vi "VisionExecute.v.vi"   [LabVIEW 2023]
uses:
  <vilib>/Rock Robotics/WPI/ThirdParty/JAS_Junk/TrajLib/Trajectory_Library.lvlib
  <vilib>/Rock Robotics/WPI/ThirdParty/PhotonVisionLib/PhotonVisionLib.lvlib
  <vilib>/Rock Robotics/WPI/ThirdParty/PhotonVisionLib/Enum/PhotonPoseStrategy_ENUM.ctl
  VisionGlobal.vi
  <vilib>/Rock Robotics/WPI/ThirdParty/JAS_Junk/TrajLib/TypeDef/TRANSLATION2D.ctl
  <vilib>/Rock Robotics/WPI/ThirdParty/JAS_Junk/TrajLib/TypeDef/ROTATION2D.ctl
  <vilib>/Rock Robotics/WPI/ThirdParty/JAS_Junk/TrajLib/TypeDef/POSE2D.ctl
  VisionNetworkingGlobal.vi
  <vilib>/Rock Robotics/Network Tables/NT Write Number.vi
  <vilib>/Rock Robotics/WPI/ThirdParty/JAS_Junk/TrajLib/VI/AprilTagFieldLayout_New2024.vi
types:
  T1 = typedef "PhotonVisionLib.lvlib/PhotonPoseStrategy_ENUM.ctl" = enum16{"LOWEST_AMBIGUITY", "CLOSEST_TO_CAMERA_HEIGHT", "CLOSEST_TO_REFERENCE_POSE", "CLOSEST_TO_LAST_POSE", "AVERAGE_BEST_TARGETS", "MULTI_TAG_PNP_ON_COPROCESSOR", "MULTI_TAG_PNP_ON_RIO"}
  T2 = typedef "Trajectory_Library.lvlib/TRANSLATION3D.ctl" = cluster{"X":dbl, "Y":dbl, "Z":dbl}
  T3 = typedef "Trajectory_Library.lvlib/ROTATION3D.ctl" = cluster{"Q_quaternion":T4}
  T4 = typedef "Trajectory_Library.lvlib/QUATERNION.ctl" = cluster{"R":dbl, "V":dbl[]}
  T5 = typedef "Trajectory_Library.lvlib/TRANSFORM3D.ctl" = cluster{"TRANSLATION3D":T2, "ROTATION3D":T3, "XF":bool}
  T6 = typedef "PhotonVisionLib.lvlib/PhotonPipelineResultType.ctl" = cluster{"Targets":T7[], "PhotonMultiTargetPNPResult":T9, "PhotonPipelineMetadata":T11}
  T7 = typedef "PhotonVisionLib.lvlib/PhotonTrackedTargetType.ctl" = cluster{"Yaw":dbl, "Pitch":dbl, "Area":dbl, "Skew":dbl, "MinAreaRectCorners":T8[], "BestCameraToTarget":T5, "FiducialId":i32, "AltCameraToTarget":T5, "PoseAmbiguity":dbl, "DetectedCorners":T8[], "ObjDetectId":i32, "ObjDetectConf":sgl}
  T8 = typedef "PhotonVisionLib.lvlib/TargetCornerType.ctl" = cluster{"X":dbl, "Y":dbl}
  T9 = typedef "PhotonVisionLib.lvlib/PhotonMultiTargetPNPResultType.ctl" = cluster{"PhotonPNPResult":T10, "FiducialIDsUsed":i16[]}
  T10 = typedef "PhotonVisionLib.lvlib/PhotonPNPResultType.ctl" = cluster{"IsPresent":bool, "bestReprojErr":dbl, "altReprojErr":dbl, "ambiguity":dbl, "Best":T5, "Alt":T5}
  T11 = typedef "PhotonVisionLib.lvlib/PhotonPipelineMetadataType.ctl" = cluster{"CaptureTimestampMicros":i64, "PublishTimestampMicros":i64, "SequenceID":i64, "TimeSinceLastPong":i64}
  T12 = typedef "Trajectory_Library.lvlib/AprilTagFieldLayout.ctl" = cluster{"AprilTagMap":map{i32, T13}, "FieldLength":dbl, "FieldWidth":dbl, "OriginPosition ":T15, "OriginPose3d":T14}
  T13 = typedef "Trajectory_Library.lvlib/AprilTag.ctl" = cluster{"ID":i32, "POSE3D":T14}
  T14 = typedef "Trajectory_Library.lvlib/POSE3D.ctl" = cluster{"Translation3d":T2, "Rotation3d":T3}
  T15 = typedef "Trajectory_Library.lvlib/AprilTagFieldLayoutOrignPosition_ENUM.ctl" = enum16{"kBlueAllianceWallRightSide,", "kRedAllianceWallRightSide,"}
  T16 = typedef "Trajectory_Library.lvlib/POSE2D.ctl" = cluster{"TRANSLATION":T17, "ROTATION":T18}
  T17 = typedef "Trajectory_Library.lvlib/TRANSLATION2D.ctl" = cluster{"X":dbl, "Y":dbl}
  T18 = typedef "Trajectory_Library.lvlib/ROTATION2D.ctl" = cluster{"VALUE":dbl, "COS":dbl, "SIN":dbl}
  T19 = typedef "PhotonVisionLib.lvlib/PhotonPoseEstimator_Configuration.ctl" = cluster{"Primary Strategy":T1, "Camera":string, "Initial Pose":T14, "HighestAmbiguity":dbl, "RobotToCamera":T5, "FallBack Strategy":T1, "BaseNTName":string}
  T20 = typedef "Trajectory_Library.lvlib/SWERVE_DRIVE_KINEMATICS.ctl" = cluster{"NumModules":i32, "InverseKinematics":T21, "ForwardKinematics":T21, "Modules":T17[], "PrevCoR":T17, "SavedModuleStates":T22[]}
  T21 = typedef "NI_Matrix.lvlib/RealMatrix.ctl" = dbl[][]
  T22 = typedef "Trajectory_Library.lvlib/SWERVE_DRIVE_MODULE_STATE.ctl" = cluster{"Speed":dbl, "Angle":T18}
  T23 = typedef "Trajectory_Library.lvlib/SWERVE_DRIVE_MODULE_POSITION.ctl" = cluster{"Distance":dbl, "Angle":T18, "P":bool}
  T24 = typedef "Trajectory_Library.lvlib/SWERVE_DRIVE_POSE_EST2_CONFIG.ctl" = cluster{"Wheel_Locations M":T17[], "Odom X std dev M":dbl, "Odom Y std dev M":dbl, "Odom Heading std dev Rad":dbl, "Vision X std dev M":dbl, "Vision Y std dev M":dbl, "Vision Heading std dev Rad":dbl}
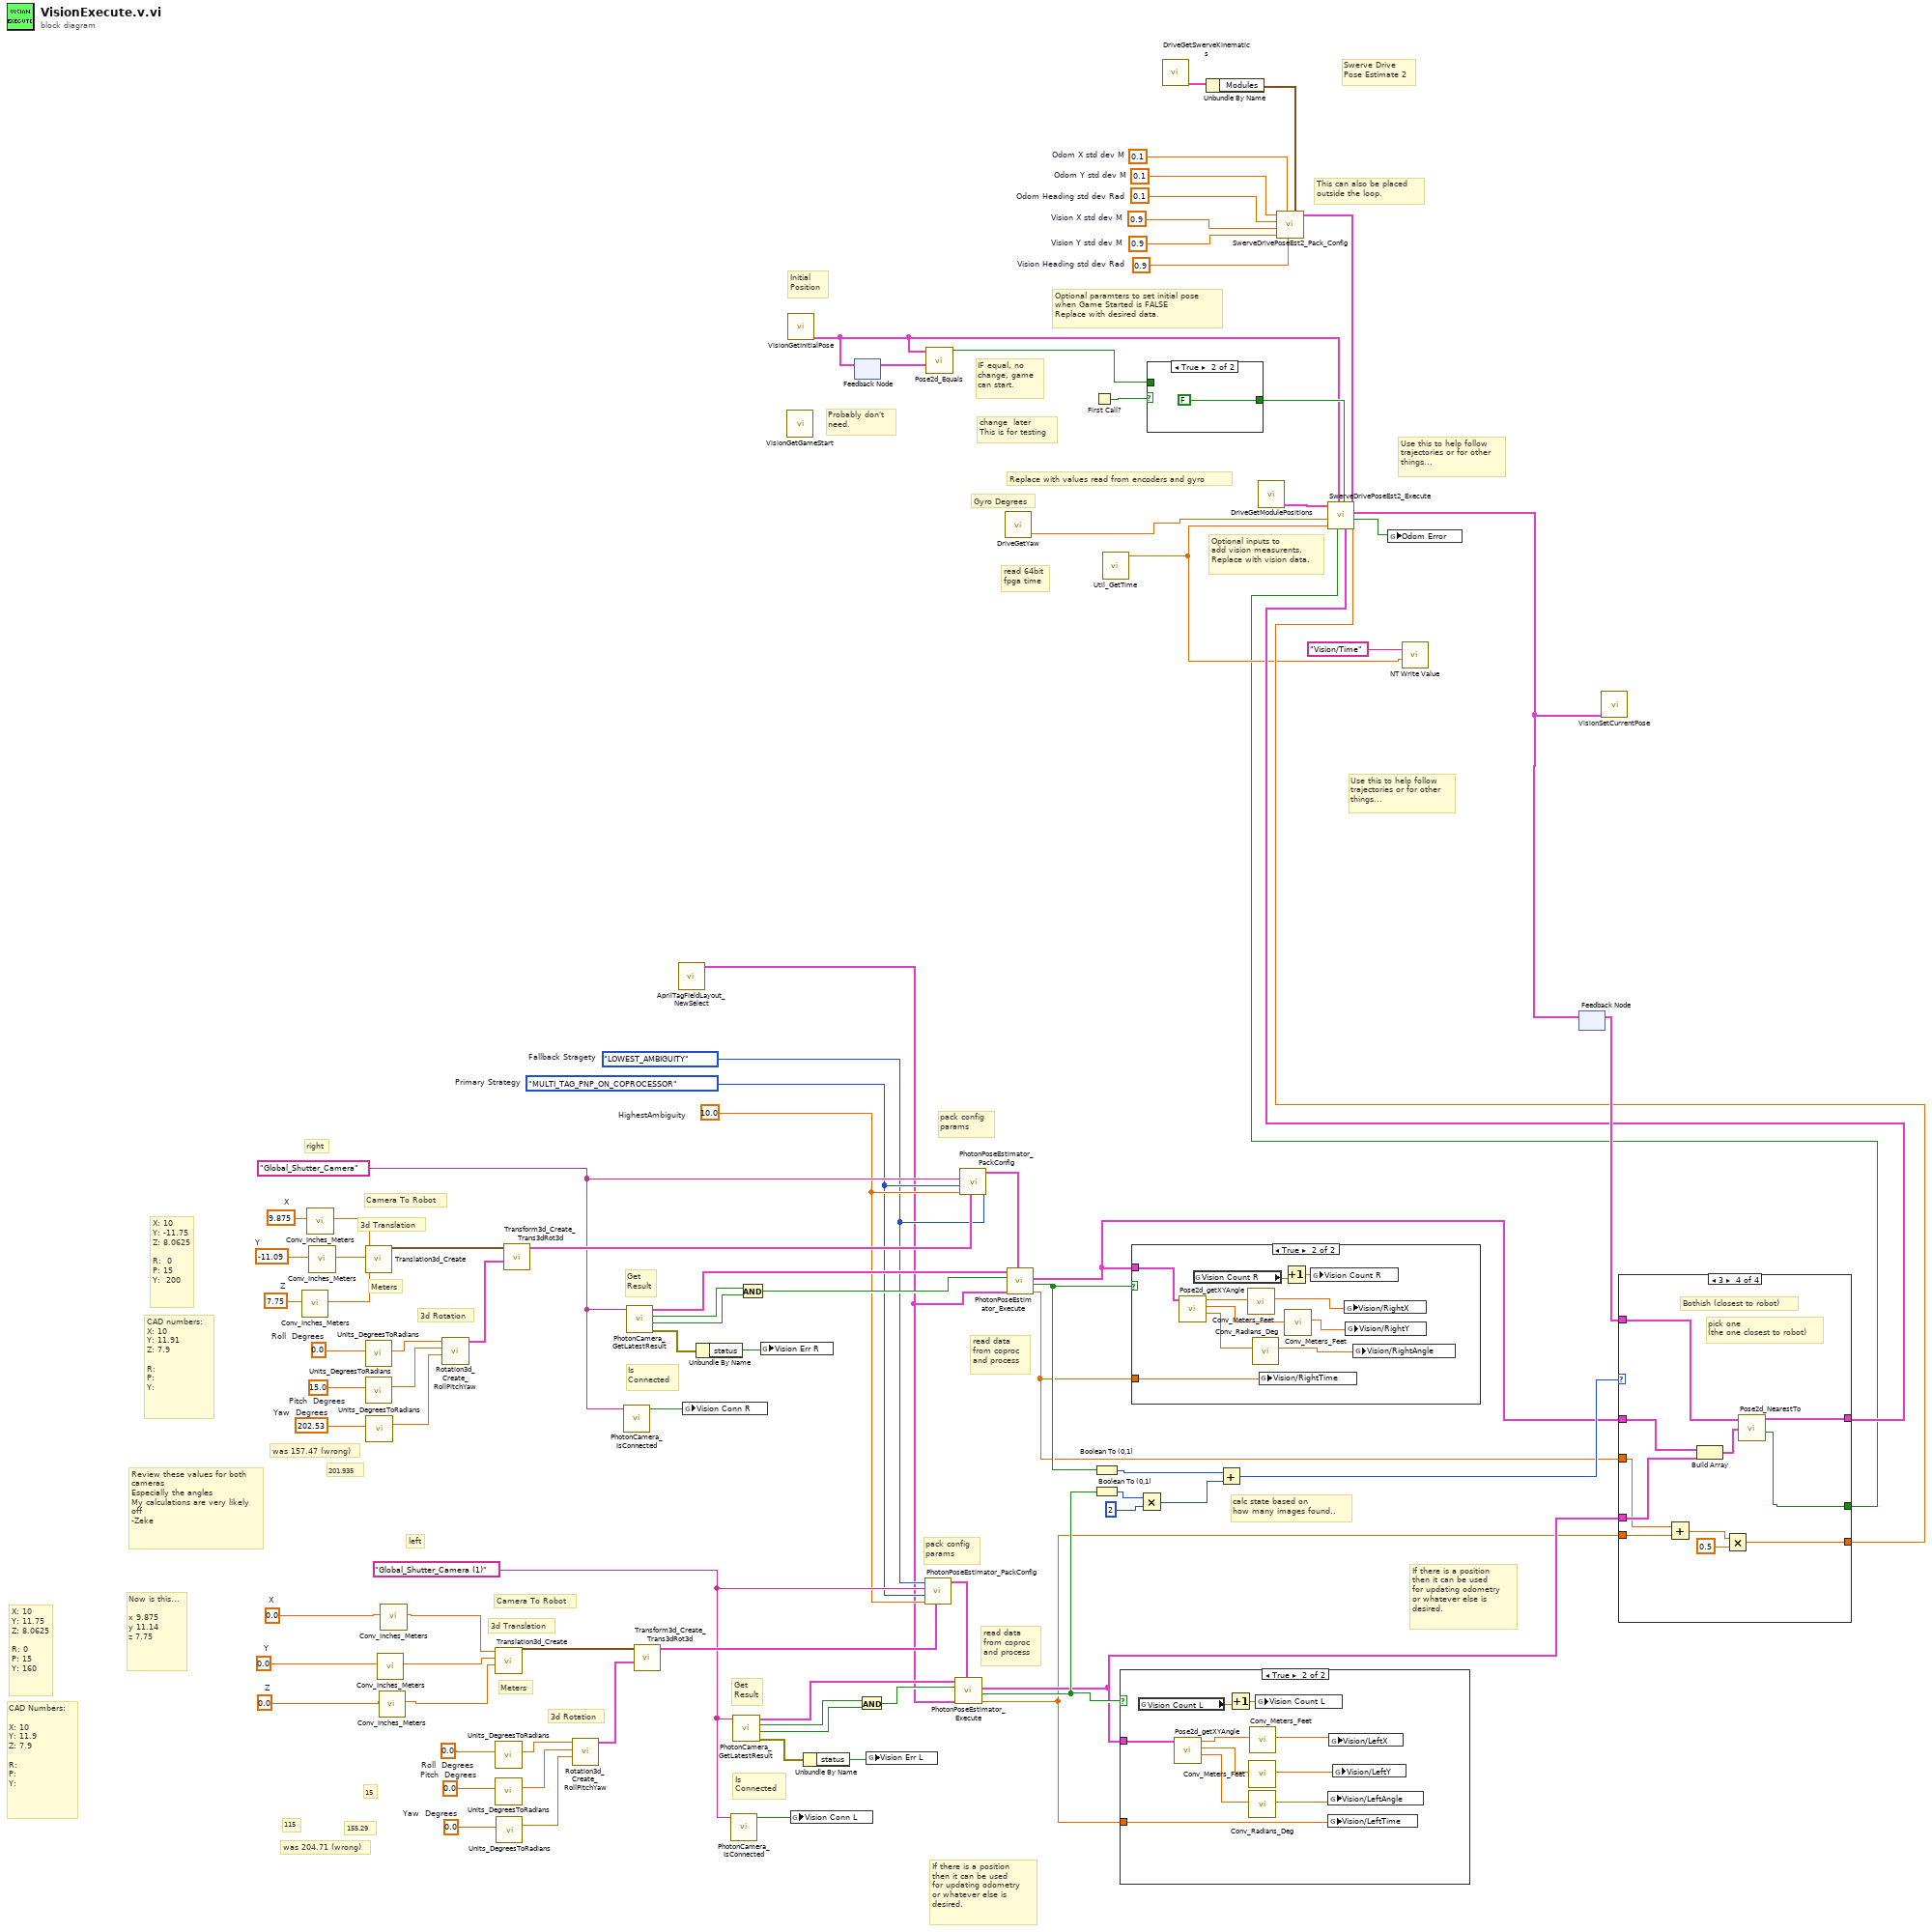
[diagram p0: block diagram]
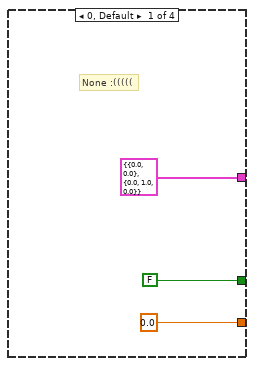
[diagram p3: hidden frame]
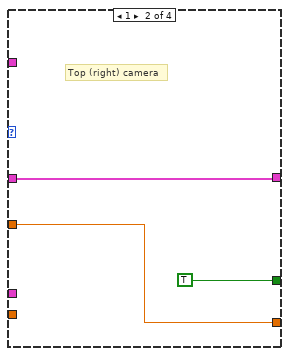
[diagram p4: hidden frame]
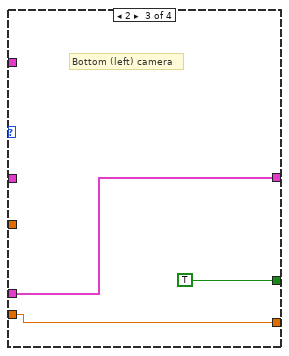
[diagram p5: hidden frame]
diagram:
  w14 = PhotonPoseStrategy_ENUM."LOWEST_AMBIGUITY"  # Fallback Stragety
  w24 = 0.1  # Odom Y std dev M
  w25 = 0.1  # Odom Heading std dev Rad
  w26 = 0.9  # Vision X std dev M
  w27 = 0.9  # Vision Y std dev M
  w28 = 0.1  # Odom X std dev M
  w29 = 0.9  # Vision Heading std dev Rad
  w62 = 0.0  # Roll  Degrees
  w61 = 0.0  # Pitch  Degrees
  w60 = 0.0  # Yaw  Degrees
  w47 = 0.0  # Z
  w51 = 0.0  # X
  w49 = 0.0  # Y
  w56 = "Global_Shutter_Camera (1)" ("CameraName")
  w80 = 0.0  # Roll  Degrees
  w79 = 15.0  # Pitch  Degrees
  w78 = 202.53  # Yaw  Degrees
  w41 = 7.75  # Z
  w45 = 9.875  # X
  w43 = -11.09  # Y
  w39 = 10.0  # HighestAmbiguity
  w38 = PhotonPoseStrategy_ENUM."MULTI_TAG_PNP_ON_COPROCESSOR"  # Primary Strategy
  w74 = "Global_Shutter_Camera" ("CameraName")
  # "calc state based on\nhow many images found.."
  # "read data\nfrom coproc\nand process"
  # "read data\nfrom coproc\nand process"
  # "pack config\nparams"
  # "pack config\nparams"
  # "15"
  # "155.29"
  # "Now is this...\n\nx 9.875\ny 11.14\nz 7.75"
  # "115"
  # "was 157.47 (wrong)"
  # "was 204.71 (wrong)"
  # "CAD Numbers:\n\nX: 10 \nY: 11.9\nZ: 7.9\n\nR:\nP:\nY:"
  # "CAD numbers:\nX: 10\nY: 11.91\nZ: 7.9\n\nR:\nP:\nY:"
  # "X: 10\nY: 11.75\nZ: 8.0625\n\nR: 0\nP: 15\nY: 160"
  # "X: 10 \nY: -11.75\nZ: 8.0625\n\nR:  0\nP: 15\nY:  200"
  # "Probably don't\nneed."
  # "IF equal, no \nchange, game\ncan start."
  # "Initial\nPosition"
  # "201.935"
  # "change  later\nThis is for testing"
  # "Review these values for both cameras\nEspecially the angles\nMy calculations are very likely off\n-Zeke"
  # "Optional inputs to\nadd vision measurents.\nReplace with vision data."
  # "Replace with values read from encoders and gyro"
  # "Optional paramters to set initial pose\nwhen Game Started is FALSE\nReplace with desired data."
  # "read 64bit\nfpga time"
  # "This can also be placed \noutside the loop."
  # "Use this to help follow\ntrajectories or for other\nthings..."
  # "Swerve Drive \nPose Estimate 2"
  # "Use this to help follow\ntrajectories or for other\nthings..."
  # "right"
  # "left"
  # "If there is a position\nthen it can be used\nfor updating odometry\nor whatever else is \ndesired."
  # "Meters"
  # "Camera To Robot"
  # "3d Rotation"
  # "3d Translation"
  # "Is\nConnected"
  # "Get\nResult"
  # "If there is a position\nthen it can be used\nfor updating odometry\nor whatever else is \ndesired."
  # "Meters"
  # "Camera To Robot"
  # "3d Rotation"
  # "3d Translation"
  # "Is\nConnected"
  # "Get\nResult"
  # "Gyro Degrees"
  n1 = call <vilib>:"Conv_Inches_Meters.vi"("INCH"=w41) -> ("Meters"=w40:dbl)  [unwired: 10 in]
  n2 = call <vilib>:"Conv_Inches_Meters.vi"("INCH"=w45) -> ("Meters"=w44:dbl)  [unwired: 10 in]
  n3 = call <vilib>:"Conv_Inches_Meters.vi"("INCH"=w43) -> ("Meters"=w42:dbl)  [unwired: 10 in]
  n4 = call <vilib>:"Translation3d_Create.vi"("Z"=w40, "Y"=w42, "X"=w44) -> ("TRANSLATION3D"=w81:T2)  [unwired: 8 in]
  n5 = call <vilib>:"Units_DegreesToRadians.vi"("Degrees"=w80) -> ("Radians"=w77:dbl)  [unwired: 10 in]
  n6 = call <vilib>:"Units_DegreesToRadians.vi"("Degrees"=w79) -> ("Radians"=w76:dbl)  [unwired: 10 in]
  n7 = call <vilib>:"Units_DegreesToRadians.vi"("Degrees"=w78) -> ("Radians"=w75:dbl)  [unwired: 10 in]
  n8 = call <vilib>:"Conv_Inches_Meters.vi"("INCH"=w49) -> ("Meters"=w48:dbl)  [unwired: 10 in]
  n9 = call <vilib>:"Conv_Inches_Meters.vi"("INCH"=w47) -> ("Meters"=w46:dbl)  [unwired: 10 in]
  n10 = call <vilib>:"Conv_Inches_Meters.vi"("INCH"=w51) -> ("Meters"=w50:dbl)  [unwired: 10 in]
  n11 = call <vilib>:"Rotation3d_Create_RollPitchYaw.vi"("Yaw"=w75, "Pitch"=w76, "Roll"=w77) -> ("Rotation3d"=w82:T3)  [unwired: 8 in]
  n12 = call <vilib>:"Translation3d_Create.vi"("Z"=w46, "Y"=w48, "X"=w50) -> ("TRANSLATION3D"=w63:T2)  [unwired: 8 in]
  n13 = call <vilib>:"Units_DegreesToRadians.vi"("Degrees"=w62) -> ("Radians"=w59:dbl)  [unwired: 10 in]
  n14 = call <vilib>:"Units_DegreesToRadians.vi"("Degrees"=w61) -> ("Radians"=w58:dbl)  [unwired: 10 in]
  n15 = call <vilib>:"Units_DegreesToRadians.vi"("Degrees"=w60) -> ("Radians"=w57:dbl)  [unwired: 10 in]
  n16 = call <vilib>:"Transform3d_Create_Trans3dRot3d.vi"("Rotation3d"=w82, "Translation3d"=w81) -> ("Transform3d"=w83:T5)  [unwired: 9 in]
  n17 = call <vilib>:"Rotation3d_Create_RollPitchYaw.vi"("Yaw"=w57, "Pitch"=w58, "Roll"=w59) -> ("Rotation3d"=w64:T3)  [unwired: 8 in]
  n18 = call <vilib>:"PhotonCamera_IsConnected.vi"("CameraName"=w74) -> ("IsConnected"=w72:bool)  [unwired: 9 in, 1 out]
  n19 = call <vilib>:"PhotonCamera_GetLatestResult.vi"("CameraName"=w74) -> ("error out"=w71:errorcluster, "New Data"=w87:bool, "HasTargets"=w86:bool, "PipelineResult"=w84:T6)  [unwired: 6 in, 1 out]
  n20 = call <vilib>:"Transform3d_Create_Trans3dRot3d.vi"("Rotation3d"=w64, "Translation3d"=w63) -> ("Transform3d"=w65:T5)  [unwired: 9 in]
  n21 = call-poly <vilib>:"AprilTagFieldLayout_NewSelect.vi"() -> ("AprilTagFieldLayout"=w1:T12)  [unwired: 11 in]
  n22 = global write "VisionGlobal.vi" "Vision Conn R"(w72) -> ()
  n23 = Unbundle By Name(w71) -> ("status"=w70:bool)
  n24 = call <vilib>:"PhotonCamera_IsConnected.vi"("CameraName"=w56) -> ("IsConnected"=w54:bool)  [unwired: 9 in, 1 out]
  n25 = call <vilib>:"PhotonCamera_GetLatestResult.vi"("CameraName"=w56) -> ("error out"=w53:errorcluster, "New Data"=w69:bool, "HasTargets"=w68:bool, "PipelineResult"=w66:T6)  [unwired: 6 in, 1 out]
  n26 = And(x=w86, y=w87) -> (x .and. y?=w85:bool)
  n27 = global write "VisionGlobal.vi" "Vision Err R"(w70) -> ()
  n28 = call "VisionGetGameStart.vi"() -> ()  [unwired: 11 in, 1 out]
  n29 = call "VisionGetInitialPose.vi"() -> ("InitialPose"=w4:T16)  [unwired: 10 in]
  n30 = global write "VisionGlobal.vi" "Vision Conn L"(w54) -> ()
  n31 = Unbundle By Name(w53) -> ("status"=w52:bool)
  n32 = feedback-in #1(w4) -> ()
  n33 = feedback #1() -> (w3:T16)  [unwired: 1 in]
  n34 = And(x=w68, y=w69) -> (x .and. y?=w67:bool)
  n35 = global write "VisionGlobal.vi" "Vision Err L"(w52) -> ()
  n36 = call <vilib>:"PhotonPoseEstimator_PackConfig.vi"("FallBack Strategy"=w14, "RobotToCamera"=w65, "HighestAmbiguity"=w39, "PirmaryStrategy"=w38, "Camera"=w56) -> ("PoseEstimator_Configuration"=w55:T19)  [unwired: 6 in]
  n37 = call <vilib>:"Pose2d_Equals.vi"("other POSE"=w3, "in POSE"=w4) -> ("Equals"=w2:bool)  [unwired: 9 in]
  n38 = call <vilib>:"PhotonPoseEstimator_Execute.vi"("Configuration"=w55, "AprilTagFieldLayout"=w1, "PIpeline Has \nNew Results"=w67, "PipelineResult"=w66) -> ("TimeStamp_Seconds"=w9:dbl, "New Pose Found"=w36:bool, "EstimatedPose2d"=w11:T16)  [unwired: 1 in, 4 out]
  n39 = call <vilib>:"PhotonPoseEstimator_PackConfig.vi"("FallBack Strategy"=w14, "RobotToCamera"=w83, "HighestAmbiguity"=w39, "PirmaryStrategy"=w38, "Camera"=w74) -> ("PoseEstimator_Configuration"=w73:T19)  [unwired: 6 in]
  n40 = call "DriveGetYaw.vi"() -> ("Yaw"=w19:dbl)  [unwired: 11 in]
  n41 = call <vilib>:"PhotonPoseEstimator_Execute.vi"("Configuration"=w73, "AprilTagFieldLayout"=w1, "PIpeline Has \nNew Results"=w85, "PipelineResult"=w84) -> ("TimeStamp_Seconds"=w8:dbl, "New Pose Found"=w37:bool, "EstimatedPose2d"=w10:T16)  [unwired: 1 in, 4 out]
  n42 = First Call?() -> (First Call?: T/F=w12:bool)
  n43 = Boolean To (0,1)(Boolean=w37) -> (0, 1=w32:i16)
  n44 = Boolean To (0,1)(Boolean=w36) -> (0, 1=w35:i16)
  n45 = call <vilib>:"Util_GetTime.vi"() -> ("FPGA_Time_Seconds"=w6:dbl)  [unwired: 9 in, 2 out]
  n46 = case shown="True" w36 {
    tunnel: w11 -> [_ w95]
    tunnel: w9 -> [_ w94]
    frame False {
    }
    frame True {
      n47 = global read "VisionGlobal.vi" "Vision Count L"() -> (w96:dbl)
      n48 = call <vilib>:"Pose2d_getXYAngle.vi"("in POSE"=w95) -> ("Angle"=w89:dbl, "Y"=w91:dbl, "X"=w93:dbl)  [unwired: 8 in]
      n49 = Increment(x=w96) -> (x+1=w97:dbl)
      n50 = call <vilib>:"Conv_Meters_Feet.vi"("Meters"=w91) -> ("Feet"=w90:dbl)  [unwired: 10 in]
      n51 = call <vilib>:"Conv_Radians_Deg.vi"("Radians"=w89) -> ("Degrees"=w88:dbl)  [unwired: 10 in]
      n52 = call <vilib>:"Conv_Meters_Feet.vi"("Meters"=w93) -> ("Feet"=w92:dbl)  [unwired: 10 in]
      n53 = global write "VisionGlobal.vi" "Vision Count L"(w97) -> ()
      n54 = global write "VisionNetworkingGlobal.vi" "Vision/LeftAngle"(w88) -> ()
      n55 = global write "VisionNetworkingGlobal.vi" "Vision/LeftTime"(w94) -> ()
      n56 = global write "VisionNetworkingGlobal.vi" "Vision/LeftX"(w92) -> ()
      n57 = global write "VisionNetworkingGlobal.vi" "Vision/LeftY"(w90) -> ()
    }
  }
  n58 = case shown="True" w37 {
    tunnel: w10 -> [_ w105]
    tunnel: w8 -> [_ w104]
    frame False {
    }
    frame True {
      n59 = call <vilib>:"Pose2d_getXYAngle.vi"("in POSE"=w105) -> ("Angle"=w99:dbl, "Y"=w101:dbl, "X"=w103:dbl)  [unwired: 8 in]
      n60 = global read "VisionGlobal.vi" "Vision Count R"() -> (w106:dbl)
      n61 = call <vilib>:"Conv_Meters_Feet.vi"("Meters"=w103) -> ("Feet"=w102:dbl)  [unwired: 10 in]
      n62 = call <vilib>:"Conv_Radians_Deg.vi"("Radians"=w99) -> ("Degrees"=w98:dbl)  [unwired: 10 in]
      n63 = global write "VisionNetworkingGlobal.vi" "Vision/RightTime"(w104) -> ()
      n64 = Increment(x=w106) -> (x+1=w107:dbl)
      n65 = call <vilib>:"Conv_Meters_Feet.vi"("Meters"=w101) -> ("Feet"=w100:dbl)  [unwired: 10 in]
      n66 = global write "VisionGlobal.vi" "Vision Count R"(w107) -> ()
      n67 = global write "VisionNetworkingGlobal.vi" "Vision/RightX"(w102) -> ()
      n68 = global write "VisionNetworkingGlobal.vi" "Vision/RightY"(w100) -> ()
      n69 = global write "VisionNetworkingGlobal.vi" "Vision/RightAngle"(w98) -> ()
    }
  }
  n70 = Multiply(x=w35, y=i16 2) -> (x*y=w33:i16)
  n71 = case shown="True" w12 {
    tunnel: [w108 FALSE] -> w13
    tunnel: w2 -> [w108 _]
    frame False {
    }
    frame True {
    }
  }
  n72 = call "DriveGetSwerveKinematics.vi"() -> ("SWERVE_DRIVE_KINEMATICS"=w16:T20)  [unwired: 11 in]
  n73 = Unbundle By Name(w16) -> ("Modules"=w15:T17[])
  n74 = Add(x=w32, y=w33) -> (x+y=w31:i16)
  n75 = call "DriveGetModulePositions.vi"() -> ("Swerve_Drive_Modual_Positions"=w20:T23[])  [unwired: 11 in]
  n76 = call <vilib>:"SwerveDrivePoseEst2_Pack_Config.vi"("Wheel_Locations M"=w15, "Vision Heading std dev Rad"=w29, "Odom X std dev M"=w28, "Vision Y std dev M"=w27, "Vision X std dev M"=w26, "Odom Heading std dev Rad"=w25, "Odom Y std dev M"=w24) -> ("SwervePoseEst2Config"=w23:T24)  [unwired: 4 in]
  n77 = call-poly <vilib>:"NT Write Value.vi"("value"=w6, "name"="Vision/Time") -> ()  [unwired: 9 in, 1 out]
  n78 = feedback #2() -> (w30:T16)  [unwired: 1 in]
  n79 = case shown="3" w31 {
    tunnel: w10 -> [_ w114 _ w127]
    tunnel: w11 -> [_ _ w117 w126]
    tunnel: w30 -> [_ _ _ w128]
    tunnel: [FALSE ("Found") TRUE ("Found") TRUE ("Found") w124] -> w5
    tunnel: w8 -> [_ w115 _ w123]
    tunnel: w9 -> [_ _ w118 w122]
    tunnel: [T16 {"TRANSLATION"={"X"=0.0, "Y"=0.0}, "ROTATION"={"VALUE"=0.0, "COS"=1.0, "SIN"=0.0}} ("Nearest Pose") w114 w117 w125] -> w18
    tunnel: [0.0 w115 w118 w119] -> w17
    frame 0, Default {
      # "None :((((("
    }
    frame 1 {
      # "Top (right) camera"
    }
    frame 2 {
      # "Bottom (left) camera"
    }
    frame 3 {
      # "pick one \n(the one closest to robot)"
      # "Bothish (closest to robot)"
      n80 = Add(x=w123, y=w122) -> (x+y=w121:dbl)
      n81 = Build Array(w127, w126) -> (w129:T16[])
      n82 = Multiply(x=w121, y=0.5) -> (x*y=w119:dbl)
      n83 = call <vilib>:"Pose2d_NearestTo.vi"("other POSE"=w129, "in POSE"=w128) -> ("Found"=w124:bool, "Nearest Pose"=w125:T16)  [unwired: 8 in]
    }
  }
  n84 = call <vilib>:"SwerveDrivePoseEst2_Execute.vi"("Vision TImeStamp_Seconds"=w17, "SwervePoseEst2Config"=w23, "visionRobotPose"=w18, "Game Started"=w13, "Add Vision Meas"=w5, "InitialPose"=w4, "Pass Through Time"=w6, "Gyro Degrees"=w19, "Module Positions"=w20) -> ("Error"=w21:bool, "Estimated Pose"=w22:T16)  [unwired: 1 in]
  n85 = global write "VisionGlobal.vi" "Odom Error"(w21) -> ()
  n86 = feedback-in #2(w22) -> ()
  n87 = call "VisionSetCurrentPose.vi"("Current Pose"=w22) -> ()  [unwired: 11 in]
